vi "Get Maximum Binning.vi"(9 "MaxBinning":i32, 10 "HorzVert":i32, 11 "ReadMode":i32) -> (1 "MaxBinning out":i32, 3 "function return":u32)   [LabVIEW 2018, in "AndorSDK.lvlib"]
doc: "EXPNETTYPE unsigned int WINAPI GetMaximumBinning(int ReadMode, int HorzVert, int * MaxBinning);"
uses:
  AndorSDK.lvlib
  ATMCD32D.dll
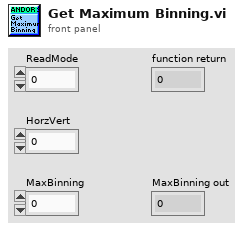
[diagram p1: front panel]
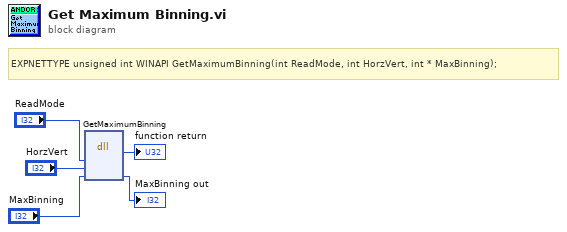
[diagram p0: block diagram]
diagram:
  # "EXPNETTYPE unsigned int WINAPI GetMaximumBinning(int ReadMode, int HorzVert, int * MaxBinning);"
  n1 = dll-call lib="PTH2babs E\nPersönliches02 - Arbeit03-HiwijobsLabviewCodelibANDOR\tAndor SDK\nATMCD32D.*" fn="GetMaximumBinning"("ReadMode"="ReadMode", "HorzVert"="HorzVert", "MaxBinning"="MaxBinning") -> (→"function return":u32, "MaxBinning"=→"MaxBinning out":i32)  [unwired: 5 in, 2 out]
